vi "close view.vi"(8 "error in (no error)":errorcluster, 11 "base view in":refnum<class "base view.lvclass">) -> (0 "error out":errorcluster, 3 "base view out":refnum<class "base view.lvclass">)   [LabVIEW 2022 SP3, in "base view.lvclass"]
uses:
  base view.lvclass
  base view.lvclass/base view.ctl
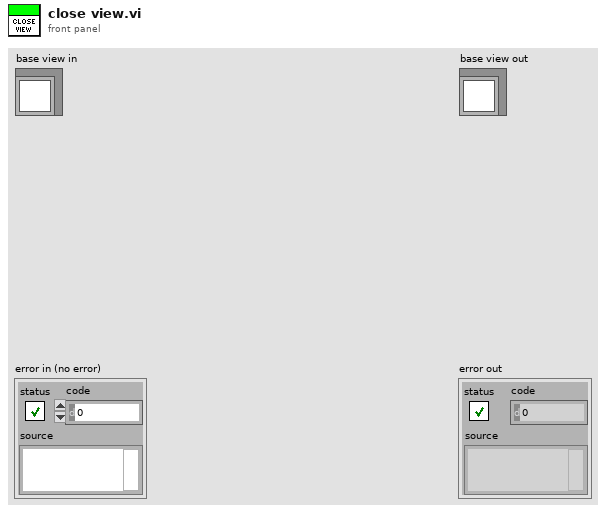
[diagram p1: front panel]
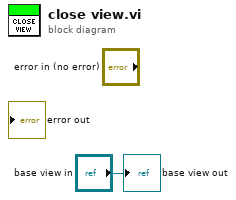
[diagram p0: block diagram]
diagram:
  "base view out" <- "base view in"
